vi "HFRR ADV v01.vi"() -> ()   [LabVIEW 2023] (continued)
                n2218 = VISA Write(VISA resource name=w3350, write buffer=w3345, error in (no error)=w3349) -> (VISA resource name out=w3348:refnum<visa-resource-name>, error out=w3347:errorcluster)  [unwired: 1 out]
              }
              frame #1 {
                n2219 = Wait (ms)(milliseconds to wait="wait") -> ()  [unwired: 1 out]
              }
              frame #2 {
                w3355 = FALSE ("Send")
                n2220 = property class="Instr"(reference=w3360, error in=w3359) -> (reference out=w3361:refnum<visa-resource-name>, error out=w3362:errorcluster, "Serial Settings:Number of Bytes at Serial Port"=w3354:u32)
                "Humidity 2" <- w3354
                n2221 = VISA Read(VISA resource name=w3361, byte count=w3354, error in (no error)=w3362) -> (VISA resource name out=w3358:refnum<visa-resource-name>, read buffer=→"Humidity Str Rec":string, error out=w3357:errorcluster)  [unwired: 1 out]
                n2222 = local write "Ser Led"(w3355) -> ()
                n2223 = local write "Send"(w3355) -> ()
              }
            }
            n2224 = Select(t=w3332, s=w3333, f=w3330) -> (s? t:f=w3331:string)
          }
        }
      }
      frame Error {
        w3378 = u16 0 items=["None"=0, "XON/XOFF"=1, "RTS/CTS"=2, "DTR/DSR"=4] ("flow control")
        w3374 = u16 0 items=["None", "Odd", "Even", "Mark", "Space"] ("parity")
        w3377 = u16 10 items=["1.0"=10, "1.5"=15, "2.0"=20] ("stop bits")
        n2225 = VISA Close(VISA resource name=w3370, error in (no error)=w3371) -> (error out=w3369:errorcluster)
        n2226 = local write "Humidity Str Rec"("" ("Humidity Str Rec")) -> ()
        n2227 = call <vilib>:"Clear Errors.vi"("error in (no error)"=w3369) -> ("error out"=w3368:errorcluster)  [unwired: 5 in, 1 out]
        n2228 = local read "Com Port 3"() -> (w3367:refnum<visa-resource-name>)
        n2229 = local write "humid"("" ("humid")) -> ()
        n2230 = call-poly "VISA Configure Serial Port"("VISA resource name"=w3367, "timeout (10sec)"=u32 1000, "termination char\n(0xA = '\\n' = LF)"=u8 10 ("termination char\n(0xA = '\\n' = LF)"), "Enable Termination\nChar (T)"=FALSE ("Enable Termination Char (T)"), "baud rate (9600)"="Humidity BaudRate", "data bits (8)"=u16 8 ("data bits"), "parity (0:none)"=w3374, "error in (no error)"=w3368, "stop bits (10: 1 bit)"=w3377, "flow control (0:none)"=w3378) -> ("VISA resource name out"=w3373:refnum<visa-resource-name>, "error out"=w3364:errorcluster)  [unwired: 4 in]
        "Port 3 Error" <- w3364
      }
    }
    n2231 = local read "Humidity Str Rec"() -> (w3265:string)
    n2232 = String Subset(string=w3265, offset (0)=7) -> (substring=w3280:string)  [unwired: 1 in]
    n2233 = Match Pattern(string=w3280, regular expression="g") -> (after substring=w3281:string, offset past match=w3272:i32)  [unwired: 1 in, 2 out]
    n2234 = Match Pattern(string=w3280, regular expression="y") -> (after substring=w3279:string, offset past match=w3273:i32)  [unwired: 1 in, 2 out]
    n2235 = Match Pattern(string=w3265, regular expression="v") -> (offset past match=w3286:i32)  [unwired: 1 in, 3 out]
    n2236 = Match Pattern(string=w3265, regular expression="?") -> (offset past match=w3283:i32)  [unwired: 1 in, 3 out]
    n2237 = Number To Decimal String(number="Set Rh") -> (decimal integer string=w3290:string)  [unwired: 1 in]
    n2238 = Greater Or Equal To 0?(x=w3273) -> (x >= 0?=w3270:bool)
    n2239 = Greater Or Equal To 0?(x=w3272) -> (x >= 0?=w3271:bool)
    n2240 = Greater Or Equal To 0?(x=w3286) -> (x >= 0?=w3268:bool)
    n2241 = Equal?(x=w3283, y=-1) -> (x = y?=w3267:bool)
    n2242 = Not Equal?(x="Set Rh", y=w3287) -> (x != y?=w3292:bool)
    n2243 = Greater?(x=w3273, y=w3272) -> (0:w3278:bool)
    n2244 = Or(x=w3270, y=w3271) -> (x .or. y?=w3269:bool)
    n2245 = Compound Arithmetic op=AND(w3268, w3267, w3269) -> (w3266:bool)
    n2246 = Concatenate Strings("#setPoint00" ("string"), w3290) -> (w3291:string)
    n2247 = Select(t=w3279, s=w3278, f=w3281) -> (s? t:f=w3274:string)
    n2248 = case shown="True" w3266 {
      tunnel: w3265 -> [_ _]
      tunnel: w3274 -> [_ w3305]
      frame False {
      }
      frame True {
        w3303 = " " ("regular expression")
        n2249 = Match Pattern(string=w3305, regular expression=" ") -> (after substring=w3307:string)  [unwired: 1 in, 3 out]
        n2250 = Match Pattern(string=w3307, regular expression=w3303) -> (before substring=→"humid":string, after substring=w3304:string)  [unwired: 1 in, 2 out]
        n2251 = Match Pattern(string=w3304, regular expression=w3303) -> (before substring=→"temp_@Rh sensor":string)  [unwired: 1 in, 3 out]
      }
    }
    n2252 = case shown="False" w3292 {
      tunnel: w3291 -> [_ w3312]
      frame False {
        n2253 = local read "Rh On/Off"() -> (w3309:bool)
        n2254 = case shown="True" w3309 {
          frame False {
            n2255 = local write "Humidity Str Send"("stop" ("Humidity Str Send")) -> ()
          }
          frame True {
            n2256 = local write "Humidity Str Send"("start" ("Humidity Str Send")) -> ()
          }
        }
      }
      frame True {
        n2257 = local write "Humidity Str Send"(w3312) -> ()
      }
    }
    n2258 = local read "EXIT"() -> (w3293:bool)
  }
  n2259 = VISA Close(VISA resource name=w8, error in (no error)=w9) -> (error out=w19:errorcluster)
  n2260 = call <vilib>:"Clear Errors.vi"("error in (no error)"=w19) -> ()  [unwired: 5 in, 2 out]
  n2261 = Or(x=w21, y=w22) -> (x .or. y?=w20:bool)
  n2262 = Or(x=w46, y=w20) -> (x .or. y?=w45:bool)
  n2263 = while {
    tunnel: [w3387] -> _
    tunnel: w16 -> [_]
    i -> [w3387]
    stop <- w3386 stop-if-true
    # "Langauage selection"
    n2264 = property on="FF Calibration g" class="WFGraph (strict)"("Plot Area:Colors:FG Color"=u32 0) -> ()  [unwired: 2 in, 2 out]
    n2265 = Equal?(x="Lan flag", y=22.0) -> ()  [unwired: 1 out]
    n2266 = case shown="True" "Case Constant\n(See Context Help) 5" {
      frame False {
      }
      frame True {
        n2267 = stacked-sequence {
          frame #0 {
            n2268 = case shown="\"Russian\"" "Language Selection" {
              tunnel: [0 1] -> w3389
              frame "English", Default {
              }
              frame "Russian" {
              }
            }
            n2269 = for {
              N: 130 -> [_]
              tunnel: "Table" -> [w3398]
              tunnel: w3389 -> [w3397]
              i -> [w3396]
              n2270 = Index Array(array=w3398, index (row)=w3396, index (col)=w3397) -> (element=w3395:string)
              n2271 = case shown="8" w3396 {
                tunnel: w3395 -> [w3399 w3400 w3401 w3402 w3403 w3404 w3405 w3406 w3407 w3408 w3409 w3410 w3411 w3412 w3413 w3414 w3415 w3416 w3417 w3418 w3419 w3420 w3421 w3422 w3423 w3424 w3425 w3426 w3427 _ _ w3428 w3429 w3430 w3431 w3432 w3433 w3442 w3449 w3456 w3463 w3467 w3470 w3473 w3475 w3477 w3478 w3479 w3480 w3481 w3482 w3483 w3484 w3485 w3486 w3487 w3488 w3489 w3490 w3491 w3492 w3493 w3494 w3495 w3496 w3497 w3498 w3499 w3500 w3501 w3502 w3503 w3504 w3505 w3506 w3507 w3508 w3509 w3510 w3511 w3512 w3513 w3514 w3515 w3516 w3517 w3518 w3519 w3520 w3521 w3522 w3523 w3524 w3525 w3526 w3527 w3528 w3529 w3530 w3531 w3532 w3533 w3534 w3535 w3536 _ w3537 w3538 w3539 w3540 w3541 w3542 w3543 w3544 w3545 w3546 w3547 w3548 w3549 _ w3550 w3551 w3552 w3553 w3554 w3555 _]
                frame 0 {
                  n2272 = local write "S"(w3399) -> ()
                }
                frame 1 {
                  n2273 = local write "S 2"(w3400) -> ()
                }
                frame 2 {
                  n2274 = property on="EXIT" class="Bool (strict)"("Boolean Text.Text"=w3401) -> ()  [unwired: 2 in, 2 out]
                }
                frame 3 {
                  n2275 = local write "S 4"(w3402) -> ()
                }
                frame 4 {
                  n2276 = property on="FILE" class="Str"("Caption.Text"=w3403) -> ()  [unwired: 2 in, 2 out]
                }
                frame 5 {
                  n2277 = property on="Fuel Discription :" class="Str"("Caption.Text"=w3404) -> ()  [unwired: 2 in, 2 out]
                }
                frame 6 {
                  n2278 = property on="Remarks :" class="Str"("Caption.Text"=w3405) -> ()  [unwired: 2 in, 2 out]
                }
                frame 7 {
                  n2279 = property on="Save & Continue" class="Bool (strict)"("Boolean Text.Text"=w3406) -> ()  [unwired: 2 in, 2 out]
                }
                frame 8 {
                  n2280 = property on="STOP 3" class="Bool (strict)"("Boolean Text.Text"=w3407) -> ()  [unwired: 2 in, 2 out]
                }
                frame 9 {
                  n2281 = property on="Set Hz" class="DigNum (strict)"("Caption.Text"=w3408) -> ()  [unwired: 2 in, 2 out]
                }
                frame 10 {
                  "String 3" <- w3409
                }
                frame 11 {
                  n2282 = property on="NORMAL LOAD" class="DigNum (strict)"("Caption.Text"=w3410) -> ()  [unwired: 2 in, 2 out]
                }
                frame 12 {
                  "String 5" <- w3411
                }
                frame 13 {
                  n2283 = property on="Set Temp" class="DigNum (strict)"("Caption.Text"=w3412) -> ()  [unwired: 2 in, 2 out]
                }
                frame 14 {
                  n2284 = local write "S 15"(w3413) -> ()
                }
                frame 15 {
                  n2285 = property on="Set Rh" class="DigNum (strict)"("Caption.Text"=w3414) -> ()  [unwired: 2 in, 2 out]
                }
                frame 16 {
                  "String 13" <- w3415
                  "String 26" <- w3415
                }
                frame 17 {
                  n2286 = local write "S 18"(w3416) -> ()
                }
                frame 18 {
                  "String 17" <- w3417
                }
                frame 19 {
                  n2287 = property on="test time" class="DigNum (strict)"("Caption.Text"=w3418) -> ()  [unwired: 2 in, 2 out]
                }
                frame 20 {
                  "String 18" <- w3419
                  "String 22" <- w3419
                }
                frame 21 {
                  n2288 = property on="Elapsed time" class="DigNum (strict)"("Caption.Text"=w3420) -> ()  [unwired: 2 in, 2 out]
                }
                frame 22 {
                  n2289 = property on="Samplingtime 2" class="DigNum (strict)"("Caption.Text"=w3421) -> ()  [unwired: 2 in, 2 out]
                }
                frame 23 {
                  "String 21" <- w3422
                }
                frame 24 {
                  n2290 = property on="Countdown" class="DigNum (strict)"("Caption.Text"=w3423) -> ()  [unwired: 2 in, 2 out]
                }
                frame 25 {
                  n2291 = property on="Countdown 2" class="DigNum (strict)"("Caption.Text"=w3424) -> ()  [unwired: 2 in, 2 out]
                }
                frame 26 {
                  n2292 = property on="Engage" class="Bool (strict)"("Boolean Text.Text"=w3425) -> ()  [unwired: 2 in, 2 out]
                }
                frame 27 {
                  n2293 = property on="Boolean  4" class="Bool (strict)"("Boolean Text.Text"=w3426) -> ()  [unwired: 2 in, 2 out]
                }
                frame 28 {
                  n2294 = property on="Test \nStatus" class="Bool (strict)"("Boolean Text.Text"=w3427) -> ()  [unwired: 2 in, 2 out]
                }
                frame 29 {
                }
                frame 30 {
                }
                frame 31 {
                  n2295 = property on="FF Calibration g" class="WFGraph (strict)"("X Scale.Name Label.Text"=w3428) -> ()  [unwired: 2 in, 2 out]
                }
                frame 32 {
                  n2296 = property on="RSTCOF" class="Bool"("Boolean Text.Text"=w3429) -> ()  [unwired: 2 in, 2 out]
                  n2297 = property on="RST FF" class="Bool"("Boolean Text.Text"=w3429) -> ()  [unwired: 2 in, 2 out]
                  n2298 = property on="RST TEMP" class="Bool"("Boolean Text.Text"=w3429) -> ()  [unwired: 2 in, 2 out]
                  n2299 = property on="RSTV1 3" class="Bool"("Boolean Text.Text"=w3429) -> ()  [unwired: 2 in, 2 out]
                  n2300 = property on="rstv2" class="Bool"("Boolean Text.Text"=w3429) -> ()  [unwired: 2 in, 2 out]
                  n2301 = property on="RSTV1 2" class="Bool"("Boolean Text.Text"=w3429) -> ()  [unwired: 2 in, 2 out]
                  n2302 = property on="RST CP" class="Bool"("Boolean Text.Text"=w3429) -> ()  [unwired: 2 in, 2 out]
                }
                frame 33 {
                  "S 61" <- w3430
                }
                frame 34 {
                  "String 23" <- w3431
                }
                frame 35 {
                  n2303 = property on="Rh Before" class="DigNum (strict)"("Caption.Text"=w3432) -> ()  [unwired: 2 in, 2 out]
                }
                frame 36 {
                  n2304 = Match Pattern(string=w3433, regular expression=",") -> (before substring=→"bs":string, after substring=→"as":string)  [unwired: 1 in, 2 out]
                  n2305 = property on="Rh After" class="DigNum (strict)"("Caption.Text"=w3433) -> ()  [unwired: 2 in, 2 out]
                }
                frame 37 {
                  n2306 = Match Pattern(string=w3442, regular expression=",") -> (before substring=w3441:string, after substring=w3440:string)  [unwired: 1 in, 2 out]
                  "bs" <- w3441
                  "as" <- w3440
                  n2307 = Concatenate Strings(w3441, w3440) -> (w3437:string)
                  n2308 = property on="Humidity before test 2" class="DigNum (strict)"("Caption.Text"=w3437) -> ()  [unwired: 2 in, 2 out]
                  n2309 = property on="Humidity before test" class="DigNum (strict)"("Caption.Text"=w3437) -> ()  [unwired: 2 in, 2 out]
                  n2310 = Concatenate Strings(w3437, "=" ("string")) -> (w3438:string)
                  n2311 = local write "S 38"(w3438) -> ()
                }
                frame 38 {
                  n2312 = Match Pattern(string=w3449, regular expression=",") -> (before substring=w3448:string, after substring=w3447:string)  [unwired: 1 in, 2 out]
                  "bs" <- w3448
                  "as" <- w3447
                  n2313 = Concatenate Strings(w3448, w3447) -> (w3444:string)
                  n2314 = property on="Humidity after test 2" class="DigNum (strict)"("Caption.Text"=w3444) -> ()  [unwired: 2 in, 2 out]
                  n2315 = Concatenate Strings(w3444, "=" ("string")) -> (w3446:string)
                  n2316 = property on="Humidity after test" class="DigNum (strict)"("Caption.Text"=w3444) -> ()  [unwired: 2 in, 2 out]
                  n2317 = local write "S 39"(w3446) -> ()
                }
                frame 39 {
                  n2318 = Match Pattern(string=w3456, regular expression=",") -> (before substring=w3455:string, after substring=w3454:string)  [unwired: 1 in, 2 out]
                  "bs" <- w3455
                  "as" <- w3454
                  n2319 = Concatenate Strings(w3455, w3454) -> (w3451:string)
                  n2320 = property on="Temperature before test 2" class="DigNum (strict)"("Caption.Text"=w3451) -> ()  [unwired: 2 in, 2 out]
                  n2321 = property on="Temperature before test" class="DigNum (strict)"("Caption.Text"=w3451) -> ()  [unwired: 2 in, 2 out]
                  n2322 = Concatenate Strings(w3451, "=" ("string")) -> (→"String 34":string)
                }
                frame 40 {
                  n2323 = Match Pattern(string=w3463, regular expression=",") -> (before substring=w3462:string, after substring=w3461:string)  [unwired: 1 in, 2 out]
                  "bs" <- w3462
                  "as" <- w3461
                  n2324 = Concatenate Strings(w3462, w3461) -> (w3458:string)
                  n2325 = property on="Temperature after test 2" class="DigNum (strict)"("Caption.Text"=w3458) -> ()  [unwired: 2 in, 2 out]
                  n2326 = Concatenate Strings(w3458, "=" ("string")) -> (→"String 35":string)
                  n2327 = property on="Temperature after test" class="DigNum (strict)"("Caption.Text"=w3458) -> ()  [unwired: 2 in, 2 out]
                }
                frame 41 {
                  n2328 = property on="AVP" class="DigNum (strict)"("Caption.Text"=w3467) -> ()  [unwired: 2 in, 2 out]
                  n2329 = property on="AVP 2" class="DigNum (strict)"("Caption.Text"=w3467) -> ()  [unwired: 2 in, 2 out]
                  n2330 = Concatenate Strings(w3467, "=" ("string")) -> (→"String 36":string)
                }
                frame 42 {
                  n2331 = property on="MWSD" class="DigNum (strict)"("Caption.Text"=w3470) -> ()  [unwired: 2 in, 2 out]
                  n2332 = property on="MWSD 2" class="DigNum (strict)"("Caption.Text"=w3470) -> ()  [unwired: 2 in, 2 out]
                  n2333 = Concatenate Strings(w3470, "=" ("string")) -> (→"String 37":string)
                }
                frame 43 {
                  n2334 = property on="HCF 2" class="DigNum (strict)"("Caption.Text"=w3473) -> ()  [unwired: 2 in, 2 out]
                  n2335 = property on="HCF" class="DigNum (strict)"("Caption.Text"=w3473) -> ()  [unwired: 2 in, 2 out]
                  n2336 = Concatenate Strings(w3473, "=" ("string")) -> (→"String 38":string)
                }
                frame 44 {
                  n2337 = Concatenate Strings(w3475, "=" ("string")) -> (→"String 39":string)
                  n2338 = property on="WS1.4 2" class="DigNum (strict)"("Caption.Text"=w3475) -> ()  [unwired: 2 in, 2 out]
                  n2339 = property on="WS1.4" class="DigNum (strict)"("Caption.Text"=w3475) -> ()  [unwired: 2 in, 2 out]
                }
                frame 45 {
                  n2340 = property on="Save Results" class="Bool (strict)"("Boolean Text.Text"=w3477) -> ()  [unwired: 2 in, 2 out]
                }
                frame 46 {
                  n2341 = local write "S 47"(w3478) -> ()
                }
                frame 47 {
                  n2342 = local write "S 48"(w3479) -> ()
                }
                frame 48 {
                  n2343 = local write "S 49"(w3480) -> ()
                }
                frame 49 {
                  n2344 = local write "S 50"(w3481) -> ()
                }
                frame 50 {
                  n2345 = local write "S 51"(w3482) -> ()
                }
                frame 51 {
                  n2346 = local write "S 52"(w3483) -> ()
                }
                frame 52 {
                  n2347 = local write "S 53"(w3484) -> ()
                }
                frame 53 {
                  n2348 = local write "S 54"(w3485) -> ()
                }
                frame 54 {
                  n2349 = local write "S 55"(w3486) -> ()
                }
                frame 55 {
                  n2350 = local write "S 56"(w3487) -> ()
                }
                frame 56 {
                  n2351 = local write "S 57"(w3488) -> ()
                }
                frame 57 {
                  n2352 = local write "S 58"(w3489) -> ()
                }
                frame 58 {
                  n2353 = local write "S 59"(w3490) -> ()
                }
                frame 59 {
                  n2354 = local write "S 60"(w3491) -> ()
                }
                frame 60 {
                  n2355 = local write "S 62"(w3492) -> ()
                }
                frame 61 {
                  n2356 = local write "S 63"(w3493) -> ()
                }
                frame 62 {
                  n2357 = local write "S 64"(w3494) -> ()
                }
                frame 63 {
                  n2358 = local write "S 65"(w3495) -> ()
                }
                frame 64 {
                  n2359 = local write "S 66"(w3496) -> ()
                }
                frame 65 {
                  n2360 = local write "S 67"(w3497) -> ()
                }
                frame 66 {
                  n2361 = local write "S 68"(w3498) -> ()
                }
                frame 67 {
                  n2362 = local write "S 69"(w3499) -> ()
                }
                frame 68 {
                  n2363 = local write "S 70"(w3500) -> ()
                }
                frame 69 {
                  n2364 = local write "S 71"(w3501) -> ()
                }
                frame 70 {
                  n2365 = local write "S 72"(w3502) -> ()
                }
                frame 71 {
                  n2366 = local write "S 73"(w3503) -> ()
                }
                frame 72 {
                  n2367 = local write "S 74"(w3504) -> ()
                }
                frame 73 {
                  n2368 = local write "S 75"(w3505) -> ()
                }
                frame 74 {
                  n2369 = local write "S 76"(w3506) -> ()
                }
                frame 75 {
                  n2370 = local write "S 77"(w3507) -> ()
                }
                frame 76 {
                  n2371 = local write "S 78"(w3508) -> ()
                }
                frame 77 {
                  n2372 = local write "S 79"(w3509) -> ()
                }
                frame 79 {
                  n2373 = property on="XY Graph 12" class="XYGraph (strict)"("Y Scale.Name Label.Text"=w3510) -> ()  [unwired: 2 in, 2 out]
                }
                frame 80 {
                  n2374 = local write "S 81"(w3511) -> ()
                  n2375 = property on="XY Graph 11" class="XYGraph (strict)"("Y Scale.Name Label.Text"=w3511) -> ()  [unwired: 2 in, 2 out]
                }
                frame 78 {
                  n2376 = property on="XY Graph 10" class="XYGraph (strict)"("X Scale.Name Label.Text"=w3512) -> ()  [unwired: 2 in, 2 out]
                  n2377 = property on="XY Graph 11" class="XYGraph (strict)"("X Scale.Name Label.Text"=w3512) -> ()  [unwired: 2 in, 2 out]
                  n2378 = property on="XY Graph 12" class="XYGraph (strict)"("X Scale.Name Label.Text"=w3512) -> ()  [unwired: 2 in, 2 out]
                  n2379 = property on="XY Graph 9" class="XYGraph (strict)"("X Scale.Name Label.Text"=w3512) -> ()  [unwired: 2 in, 2 out]
                }
                frame 81 {
                  n2380 = property on="XY Graph 10" class="XYGraph (strict)"("Y Scale.Name Label.Text"=w3513) -> ()  [unwired: 2 in, 2 out]
                }
                frame 82 {
                  n2381 = local write "S 84"(w3514) -> ()
                }
                frame 83 {
                  n2382 = local write "S 85"(w3515) -> ()
                }
                frame 84 {
                  n2383 = local write "S 86"(w3516) -> ()
                }
                frame 85 {
                  n2384 = local write "S 87"(w3517) -> ()
                }
                frame 86 {
                  n2385 = local write "S 88"(w3518) -> ()
                }
                frame 87 {
                  n2386 = property on="FF Calibration g" class="WFGraph (strict)"("Y Scale.Name Label.Text"=w3519) -> ()  [unwired: 2 in, 2 out]
                }
                frame 88 {
                  n2387 = local write "S 90"(w3520) -> ()
                }
                frame 89 {
                  n2388 = local write "S 91"(w3521) -> ()
                }
                frame 90 {
                  n2389 = local write "S 92"(w3522) -> ()
                }
                frame 91 {
                  n2390 = local write "S 93"(w3523) -> ()
                }
                frame 92 {
                  n2391 = local write "S 94"(w3524) -> ()
                }
                frame 93 {
                  n2392 = local write "S 95"(w3525) -> ()
                }
                frame 94 {
                  n2393 = local write "S 96"(w3526) -> ()
                }
                frame 95 {
                  n2394 = local write "S 97"(w3527) -> ()
                }
                frame 96 {
                  n2395 = local write "S 98"(w3528) -> ()
                }
                frame 97 {
                  n2396 = local write "S 99"(w3529) -> ()
                }
                frame 98 {
                  n2397 = local write "S 100"(w3530) -> ()
                }
                frame 99 {
                  n2398 = local write "S 101"(w3531) -> ()
                }
                frame 100 {
                  n2399 = local write "S 102"(w3532) -> ()
                }
                frame 101 {
                  n2400 = local write "S 103"(w3533) -> ()
                }
                frame 102 {
                  n2401 = local write "S 104"(w3534) -> ()
                }
                frame 103 {
                  n2402 = local write "S 105"(w3535) -> ()
                }
                frame 104 {
                  n2403 = local write "S 106"(w3536) -> ()
                }
                frame 105 {
                }
                frame 106 {
                  n2404 = property on="OK Button 17" class="Bool (strict)"("Boolean Text.Text"=w3537) -> ()  [unwired: 2 in, 2 out]
                }
                frame 107 {
                  n2405 = property on="OK Button 16" class="Bool (strict)"("Boolean Text.Text"=w3538) -> ()  [unwired: 2 in, 2 out]
                }
                frame 108 {
                  n2406 = property on="TITTLE" class="Str"("Caption.Text"=w3539) -> ()  [unwired: 2 in, 2 out]
                }
                frame 109 {
                  "String 30" <- w3540
                }
                frame 110 {
                  n2407 = property on="Test Date" class="Str"("Caption.Text"=w3541) -> ()  [unwired: 2 in, 2 out]
                  "String 31" <- w3541
                }
                frame 111 {
                  n2408 = property on="Sample ID" class="Str"("Caption.Text"=w3542) -> ()  [unwired: 2 in, 2 out]
                  "String 32" <- w3542
                }
                frame 112 {
                  n2409 = property on="Tested by" class="Str"("Caption.Text"=w3543) -> ()  [unwired: 2 in, 2 out]
                  "String 33" <- w3543
                }
                frame 113 {
                  n2410 = property on="System Configured Printers 2" class="Arr (strict)"("Caption.Text"=w3544) -> ()  [unwired: 2 in, 2 out]
                }
                frame 114 {
                  n2411 = property on="Selected Printer" class="Str"("Caption.Text"=w3545) -> ()  [unwired: 2 in, 2 out]
                }
                frame 115 {
                  n2412 = property on="Select Printer 3" class="DigNum (strict)"("Caption.Text"=w3546) -> ()  [unwired: 2 in, 2 out]
                }
                frame 116 {
                  n2413 = property on="Print" class="Bool (strict)"("Boolean Text.Text"=w3547) -> ()  [unwired: 2 in, 2 out]
                }
                frame 117 {
                  "String 41" <- w3548
                }
                frame 118 {
                  n2414 = property on="tested by" class="Str"("Caption.Text"=w3549) -> ()  [unwired: 2 in, 2 out]
                }
                frame 119 {
                }
                frame 120 {
                  n2415 = property on="Export" class="Bool (strict)"("Boolean Text.Text"=w3550) -> ()  [unwired: 2 in, 2 out]
                }
                frame 121 {
                  n2416 = property on="TEMP INTERCEPT:" class="DigNum (strict)"("Caption.Text"=w3551) -> ()  [unwired: 2 in, 2 out]
                }
                frame 122 {
                  n2417 = property on="AIR TEMP INTERCEPT:" class="DigNum (strict)"("Caption.Text"=w3552) -> ()  [unwired: 2 in, 2 out]
                }
                frame 123 {
                  n2418 = property on="Select File Type" class="Enum (strict)"("Caption.Text"=w3553) -> ()  [unwired: 2 in, 2 out]
                }
                frame 124 {
                  n2419 = property on="s.NO" class="Str"("Caption.Text"=w3554) -> ()  [unwired: 2 in, 2 out]
                  "String 45" <- w3554
                }
                frame 125 {
                  n2420 = property on="trip1 8" class="Bool (strict)"("Boolean Text.Text"=w3555) -> ()  [unwired: 2 in, 2 out]
                }
                frame 126, Default {
                }
              }
            }
          }
          frame #1 {
            w3563 = TRUE ("Visible")
            n2421 = local read "S 91"() -> (w3580:string)
            n2422 = local read "S 90"() -> (w3579:string)
            n2423 = local read "S 88"() -> (w3578:string)
            n2424 = property on="Threshold" class="DigNum (strict)"("Caption.Text"=w3580) -> ()  [unwired: 2 in, 2 out]
            n2425 = property on="File Path" class="Path"("Caption.Text"=w3579) -> ()  [unwired: 2 in, 2 out]
            n2426 = property on="SrvM CP" class="Bool (strict)"("Boolean Text.Text"=w3578) -> ()  [unwired: 2 in, 2 out]
            n2427 = local read "S 71"() -> (w3573:string)
            n2428 = local read "S 86"() -> (w3575:string)
            n2429 = local read "S 85"() -> (w3576:string)
            n2430 = local read "S 87"() -> (w3574:string)
            n2431 = local read "S 84"() -> (w3577:string)
            n2432 = local read "S 103"() -> (w3562:string)
            n2433 = local read "S 104"() -> (w3561:string)
            n2434 = property on="ENTER THE NEW PASSWORD" class="Str"("Caption.Text"=w3574) -> ()  [unwired: 2 in, 2 out]
            n2435 = property on="Password" class="Str"("Caption.Text"=w3576) -> ()  [unwired: 2 in, 2 out]
            n2436 = property on="ENTER CURRENT PASSWORD" class="Str"("Caption.Text"=w3575) -> ()  [unwired: 2 in, 2 out]
            n2437 = property on="EDIT" class="Bool (strict)"("Boolean Text.Text"=w3573) -> ()  [unwired: 2 in, 2 out]
            n2438 = property on="SAVE" class="Bool (strict)"("Boolean Text.Text"=w3577) -> ()  [unwired: 2 in, 2 out]
            n2439 = Build Array(w3562, w3561) -> (w3560:string[])
            n2440 = property on="Heater Button" class="Bool (strict)"("Strings [4]"=w3560) -> ()  [unwired: 2 in, 2 out]
            n2441 = property on="CH-HUMIDITY WET" class="DigNum (strict)"("Caption.Size to Text?"=w3563) -> ()  [unwired: 2 in, 2 out]
            n2442 = property on="CH-HUMIDITY DRY" class="DigNum (strict)"("Caption.Size to Text?"=w3563) -> ()  [unwired: 2 in, 2 out]
            n2443 = property on="CH-POWER -" class="DigNum (strict)"("Caption.Size to Text?"=w3563) -> ()  [unwired: 2 in, 2 out]
            n2444 = property on="CH-HEATER" class="DigNum (strict)"("Caption.Size to Text?"=w3563) -> ()  [unwired: 2 in, 2 out]
            n2445 = property on="CH-POWER +" class="DigNum (strict)"("Caption.Size to Text?"=w3563) -> ()  [unwired: 2 in, 2 out]
            n2446 = local read "S 92"() -> (w3572:string)
            n2447 = local read "S 93"() -> (w3571:string)
            n2448 = local read "S 105"() -> (w3558:string)
            n2449 = local read "S 106"() -> (w3557:string)
            n2450 = Build Array(w3572, w3571) -> ()  [unwired: 1 out]
            n2451 = Build Array(w3558, w3557) -> (w3559:string[])
            n2452 = local read "S 95"() -> (w3569:string)
            n2453 = local read "S 94"() -> (w3570:string)
            n2454 = local read "bs"() -> (w3585:string)
            n2455 = local read "as"() -> (w3586:string)
            n2456 = property on="Rh On/Off" class="Bool (strict)"("Strings [4]"=w3559) -> ()  [unwired: 2 in, 2 out]
            n2457 = Concatenate Strings(w3585, "\r", w3586) -> ()  [unwired: 1 out]
            n2458 = property on="STROKE GAIN :" class="DigNum (strict)"("Caption.Text"=w3569) -> ()  [unwired: 2 in, 2 out]
            n2459 = property on="DISPLACEMENT :" class="DigNum (strict)"("Caption.Text"=w3570) -> ()  [unwired: 2 in, 2 out]
            n2460 = property on="Rh After" class="DigNum (strict)"("Caption.Size to Text?"=TRUE ("Caption.Size to Text")) -> ()  [unwired: 2 in, 2 out]
            n2461 = local read "S 48"() -> (w3609:string)
            n2462 = local read "S 50"() -> (w3607:string)
            n2463 = local read "S 51"() -> (w3606:string)
            n2464 = local read "S 49"() -> (w3608:string)
            n2465 = local read "S 52"() -> (w3605:string)
            n2466 = local read "as"() -> (w3590:string)
            n2467 = local read "bs"() -> (w3591:string)
            n2468 = local read "S 56"() -> (w3604:string)
            n2469 = local read "S 57"() -> (w3603:string)
            n2470 = local read "S 58"() -> (w3602:string)
            n2471 = local read "S 59"() -> (w3601:string)
            n2472 = property on="OPEN" class="Bool (strict)"("Boolean Text.Text"=w3605) -> ()  [unwired: 2 in, 2 out]
            n2473 = property on="OPEN 1" class="Bool (strict)"("Boolean Text.Text"=w3609) -> ()  [unwired: 2 in, 2 out]
            n2474 = property on="OPEN 2" class="Bool (strict)"("Boolean Text.Text"=w3608) -> ()  [unwired: 2 in, 2 out]
            n2475 = property on="OPEN 3" class="Bool (strict)"("Boolean Text.Text"=w3607) -> ()  [unwired: 2 in, 2 out]
            n2476 = property on="OPEN 4" class="Bool (strict)"("Boolean Text.Text"=w3606) -> ()  [unwired: 2 in, 2 out]
            n2477 = Concatenate Strings(w3591, "\r", w3590) -> ()  [unwired: 1 out]
            n2478 = local read "S 102"() -> (w3564:string)
            n2479 = property on="КОФ1" class="DigNum (strict)"("Caption.Text"=w3604) -> ()  [unwired: 2 in, 2 out]
            n2480 = local read "S 98"() -> (w3568:string)
            n2481 = local read "S 99"() -> (w3567:string)
            n2482 = local read "S 100"() -> (w3566:string)
            n2483 = local read "S 101"() -> (w3565:string)
            n2484 = property on="КОФ2" class="DigNum (strict)"("Caption.Text"=w3603) -> ()  [unwired: 2 in, 2 out]
            n2485 = property on="КОФ3" class="DigNum (strict)"("Caption.Text"=w3602) -> ()  [unwired: 2 in, 2 out]
            n2486 = property on="КОФ4" class="DigNum (strict)"("Caption.Text"=w3601) -> ()  [unwired: 2 in, 2 out]
            n2487 = local read "bs"() -> (w3589:string)
            n2488 = local read "as"() -> (w3588:string)
            n2489 = property on="CH-POWER +" class="DigNum (strict)"("Caption.Text"=w3568) -> ()  [unwired: 2 in, 2 out]
            n2490 = property on="CH-POWER -" class="DigNum (strict)"("Caption.Text"=w3567) -> ()  [unwired: 2 in, 2 out]
            n2491 = property on="CH-HEATER" class="DigNum (strict)"("Caption.Text"=w3566) -> ()  [unwired: 2 in, 2 out]
            n2492 = property on="CH-HUMIDITY DRY" class="DigNum (strict)"("Caption.Text"=w3565) -> ()  [unwired: 2 in, 2 out]
            n2493 = property on="CH-HUMIDITY WET" class="DigNum (strict)"("Caption.Text"=w3564) -> ()  [unwired: 2 in, 2 out]
            n2494 = local read "S 60"() -> (w3600:string)
            n2495 = local read "S 54"() -> (w3610:string)
            n2496 = Concatenate Strings(w3589, "\r", w3588) -> ()  [unwired: 1 out]
            n2497 = Concatenate Strings(w3610, w3600) -> ()  [unwired: 1 out]
            n2498 = local read "S 77"() -> (→"String 43":string)
            n2499 = local read "S 76"() -> (w3583:string)
            n2500 = local read "S 78"() -> (w3582:string)
            n2501 = local read "S 71"() -> (w3594:string)
            n2502 = local read "S 66"() -> (w3599:string)
            n2503 = local read "S 67"() -> (w3598:string)
            n2504 = local read "S 68"() -> (w3597:string)
            n2505 = local read "S 69"() -> (w3596:string)
            n2506 = local read "S 70"() -> (w3595:string)
            n2507 = property on="AIR TEMP" class="DigNum (strict)"("Caption.Text"=w3582) -> ()  [unwired: 2 in, 2 out]
            n2508 = property on="Set Strk" class="DigNum (strict)"("Caption.Text"=w3583) -> ()  [unwired: 2 in, 2 out]
            n2509 = property on="FRIC. FORCE :" class="DigNum (strict)"("Caption.Text"=w3599) -> ()  [unwired: 2 in, 2 out]
            n2510 = property on="TEMPERATURE :" class="DigNum (strict)"("Caption.Text"=w3598) -> ()  [unwired: 2 in, 2 out]
            n2511 = property on="SPEED OUT:" class="DigNum (strict)"("Caption.Text"=w3597) -> ()  [unwired: 2 in, 2 out]
            n2512 = property on="AIR TEMPERATURE :" class="DigNum (strict)"("Caption.Text"=w3596) -> ()  [unwired: 2 in, 2 out]
            n2513 = property on="HUMIDITY:" class="DigNum (strict)"("Caption.Text"=w3595) -> ()  [unwired: 2 in, 2 out]
            n2514 = property on="EDIT" class="Bool (strict)"("Boolean Text.Text"=w3594) -> ()  [unwired: 2 in, 2 out]
            n2515 = local read "S 79"() -> (w3581:string)
            n2516 = property on="Stroke" class="DigNum (strict)"("Caption.Text"=w3581) -> ()  [unwired: 2 in, 2 out]
          }
          frame #2 {
          }
        }
        n2517 = local write "Lan flag"(10.0 ("Lan flag")) -> ()
      }
    }
    n2518 = Wait (ms)(milliseconds to wait=u32 50) -> ()  [unwired: 1 out]
    n2519 = local read "EXIT"() -> (w3386:bool)
  }
  n2520 = flat-sequence {
    tunnel: w43 -> [_]
    frame #0 {
    }
    frame #1 {
      n2521 = Quit LabVIEW(quit? (T)=TRUE) -> ()
      n2522 = local write "EXIT"(FALSE ("EXIT")) -> ()
    }
  }
  n2523 = while {
    tunnel: [w3620] -> w41
    i -> [w3619]
    stop <- w3620 stop-if-true
    n2524 = local read "EXIT"() -> (w3620:bool)
    n2525 = Equal To 0?(x=w3619) -> (x = 0?=w3617:bool)
    n2526 = call "Elapsed Time3"("Time Target (s)"=45.0, "Auto Reset"=TRUE) -> ("Time has Elapsed"=w3616:bool)  [unwired: 10 in, 7 out]
    n2527 = Wait (ms)(milliseconds to wait=u32 50) -> ()  [unwired: 1 out]
    n2528 = Or(x=w3616, y=w3617) -> (x .or. y?=w3618:bool)
    n2529 = case shown="True" w3618 {
      frame False {
      }
      frame True {
        n2530 = call <vilib>:"System Exec.vi"("run minimized? (F)"=TRUE, "error in (no error)"="error in (no error)", "command line"="powercfg.exe -change -monitor-timeout-ac 0") -> ("error out"=w3631:errorcluster)  [unwired: 5 in, 3 out]
        n2531 = call <vilib>:"System Exec.vi"("run minimized? (F)"=TRUE, "error in (no error)"=w3631, "command line"="powercfg.exe -change -disk-timeout-ac 0") -> ("error out"=w3630:errorcluster)  [unwired: 5 in, 3 out]
        n2532 = call <vilib>:"System Exec.vi"("run minimized? (F)"=TRUE, "error in (no error)"=w3630, "command line"="powercfg.exe -change -standby-timeout-ac 0") -> ("error out"=w3629:errorcluster)  [unwired: 5 in, 3 out]
        n2533 = call <vilib>:"System Exec.vi"("run minimized? (F)"=TRUE, "error in (no error)"=w3629, "command line"="powercfg.exe -change -hibernate-timeout-ac 0") -> ("error out"=w3628:errorcluster)  [unwired: 5 in, 3 out]
        n2534 = call <vilib>:"Simple Error Handler.vi"("error in (no error)"=w3628) -> ("error out"=w3634:errorcluster)  [unwired: 4 in, 4 out]
        n2535 = call <vilib>:"Clear Errors.vi"("error in (no error)"=w3634) -> ("error out"=→"error out":errorcluster)  [unwired: 5 in, 1 out]
      }
    }
  }
  n2536 = Compound Arithmetic op=OR(w44, w45, w41) -> (w43:bool)
  n2537 = case shown="True" "Case Constant\n(See Context Help) 6" {
    tunnel: w16 -> [_ w3636]
    frame False {
    }
    frame True {
      n2538 = while {
        tunnel: w3636 -> [_]
        tunnel: [w3637] -> _
        i -> [w3637]
        stop <- w3638 continue-if-true
        n2539 = Wait (ms)(milliseconds to wait=u32 50) -> ()  [unwired: 1 out]
        n2540 = stacked-sequence {
          frame #0 {
            # "Controls Text color"
            # "Controls BG color"
            n2541 = property on="FILE" class="Str"("Text.Text Colors:Text Color"="SC  Text") -> ()  [unwired: 2 in, 2 out]
            n2542 = property on="Fuel Discription :" class="Str"("Text.Text Colors:Text Color"="SC  Text") -> ()  [unwired: 2 in, 2 out]
            n2543 = property on="tested by" class="Str"("Text.Text Colors:Text Color"="SC  Text") -> ()  [unwired: 2 in, 2 out]
            n2544 = property on="Remarks :" class="Str"("Text.Text Colors:Text Color"="SC  Text") -> ()  [unwired: 2 in, 2 out]
            n2545 = property class="DigNum (strict)"("Numeric Text.Text Colors:BG Color"="NC BG") -> ()  [unwired: 2 in, 2 out]
            n2546 = property class="DigNum (strict)"("Numeric Text.Text Colors:BG Color"="NC BG") -> ()  [unwired: 2 in, 2 out]
            n2547 = property class="DigNum (strict)"("Numeric Text.Text Colors:BG Color"="NC BG") -> ()  [unwired: 2 in, 2 out]
            n2548 = property class="DigNum (strict)"("Numeric Text.Text Colors:BG Color"="NC BG") -> ()  [unwired: 2 in, 2 out]
            n2549 = property class="DigNum (strict)"("Numeric Text.Text Colors:BG Color"="NC BG") -> ()  [unwired: 2 in, 2 out]
            n2550 = property class="DigNum (strict)"("Numeric Text.Text Colors:BG Color"="NC BG") -> ()  [unwired: 2 in, 2 out]
            n2551 = property class="DigNum (strict)"("Numeric Text.Text Colors:BG Color"="NC BG") -> ()  [unwired: 2 in, 2 out]
            n2552 = property class="DigNum (strict)"("Numeric Text.Text Colors:BG Color"="NC BG") -> ()  [unwired: 2 in, 2 out]
            n2553 = property class="DigNum (strict)"("Numeric Text.Text Colors:BG Color"="NC BG") -> ()  [unwired: 2 in, 2 out]
            n2554 = property class="DigNum (strict)"("Numeric Text.Text Colors:BG Color"="NC BG") -> ()  [unwired: 2 in, 2 out]
            n2555 = property class="DigNum (strict)"("Numeric Text.Text Colors:BG Color"="NC BG") -> ()  [unwired: 2 in, 2 out]
            n2556 = property class="DigNum (strict)"("Numeric Text.Text Colors:BG Color"="NC BG") -> ()  [unwired: 2 in, 2 out]
            n2557 = property on="FILE" class="Str"("Text.Text Colors:BG Color"="SC BG 3") -> ()  [unwired: 2 in, 2 out]
            n2558 = property on="Fuel Discription :" class="Str"("Text.Text Colors:BG Color"="SC BG 3") -> ()  [unwired: 2 in, 2 out]
            n2559 = property on="tested by" class="Str"("Text.Text Colors:BG Color"="SC BG 3") -> ()  [unwired: 2 in, 2 out]
            n2560 = property on="Remarks :" class="Str"("Text.Text Colors:BG Color"="SC BG 3") -> ()  [unwired: 2 in, 2 out]
            n2561 = property class="DigNum (strict)"("Numeric Text.Text Colors:Text Color"="NC Text") -> ()  [unwired: 2 in, 2 out]
            n2562 = property class="DigNum (strict)"("Numeric Text.Text Colors:Text Color"="NC Text") -> ()  [unwired: 2 in, 2 out]
            n2563 = property class="DigNum (strict)"("Numeric Text.Text Colors:Text Color"="NC Text") -> ()  [unwired: 2 in, 2 out]
            n2564 = property class="DigNum (strict)"("Numeric Text.Text Colors:Text Color"="NC Text") -> ()  [unwired: 2 in, 2 out]
            n2565 = property class="DigNum (strict)"("Numeric Text.Text Colors:Text Color"="NC Text") -> ()  [unwired: 2 in, 2 out]
            n2566 = property class="DigNum (strict)"("Numeric Text.Text Colors:Text Color"="NC Text") -> ()  [unwired: 2 in, 2 out]
            n2567 = property class="DigNum (strict)"("Numeric Text.Text Colors:Text Color"="NC Text") -> ()  [unwired: 2 in, 2 out]
            n2568 = property class="DigNum (strict)"("Numeric Text.Text Colors:Text Color"="NC Text") -> ()  [unwired: 2 in, 2 out]
            n2569 = property class="DigNum (strict)"("Numeric Text.Text Colors:Text Color"="NC Text") -> ()  [unwired: 2 in, 2 out]
            n2570 = property class="DigNum (strict)"("Numeric Text.Text Colors:Text Color"="NC Text") -> ()  [unwired: 2 in, 2 out]
            n2571 = property class="DigNum (strict)"("Numeric Text.Text Colors:Text Color"="NC Text") -> ()  [unwired: 2 in, 2 out]
            n2572 = property class="DigNum (strict)"("Numeric Text.Text Colors:Text Color"="NC Text") -> ()  [unwired: 2 in, 2 out]
            n2573 = property class="DigNum (strict)"("Numeric Text.Text Colors:Text Color"="NI Text  2") -> ()  [unwired: 2 in, 2 out]
            n2574 = property class="DigNum (strict)"("Numeric Text.Text Colors:Text Color"="NI Text  2") -> ()  [unwired: 2 in, 2 out]
            n2575 = property class="DigNum (strict)"("Numeric Text.Text Colors:Text Color"="NI Text  2") -> ()  [unwired: 2 in, 2 out]
            n2576 = property class="DigNum (strict)"("Numeric Text.Text Colors:Text Color"="NI Text  2") -> ()  [unwired: 2 in, 2 out]
            n2577 = property class="DigNum (strict)"("Numeric Text.Text Colors:Text Color"="NI Text  2") -> ()  [unwired: 2 in, 2 out]
            n2578 = property class="DigNum (strict)"("Numeric Text.Text Colors:Text Color"="NI Text  2") -> ()  [unwired: 2 in, 2 out]
            n2579 = property class="DigNum (strict)"("Numeric Text.Text Colors:Text Color"="NI Text  2") -> ()  [unwired: 2 in, 2 out]
            n2580 = property class="DigNum (strict)"("Numeric Text.Text Colors:Text Color"="NI Text  2") -> ()  [unwired: 2 in, 2 out]
            n2581 = property class="DigNum (strict)"("Numeric Text.Text Colors:Text Color"="NI Text  2") -> ()  [unwired: 2 in, 2 out]
            n2582 = property class="DigNum (strict)"("Numeric Text.Text Colors:Text Color"="NI Text  2") -> ()  [unwired: 2 in, 2 out]
            n2583 = property class="DigNum (strict)"("Numeric Text.Text Colors:Text Color"="NI Text  2") -> ()  [unwired: 2 in, 2 out]
            n2584 = property class="DigNum (strict)"("Numeric Text.Text Colors:Text Color"="NI Text  2") -> ()  [unwired: 2 in, 2 out]
            n2585 = property class="DigNum (strict)"("Numeric Text.Text Colors:Text Color"="NI Text  2") -> ()  [unwired: 2 in, 2 out]
            n2586 = property class="DigNum (strict)"("Numeric Text.Text Colors:Text Color"="NI Text  2") -> ()  [unwired: 2 in, 2 out]
            n2587 = property class="DigNum (strict)"("Numeric Text.Text Colors:Text Color"="NI Text  2") -> ()  [unwired: 2 in, 2 out]
            n2588 = property class="DigNum (strict)"("Numeric Text.Text Colors:Text Color"="NI Text  2") -> ()  [unwired: 2 in, 2 out]
            n2589 = property on="XY Graph 9" class="XYGraph (strict)"("Plot Area:Colors:FG Color"="GFG  2", "Plot Area:Colors:BG Color"="GBG   2") -> ()  [unwired: 2 in, 2 out]
            n2590 = property on="XY Graph 11" class="XYGraph (strict)"("Plot Area:Colors:FG Color"="GFG  2", "Plot Area:Colors:BG Color"="GBG   2") -> ()  [unwired: 2 in, 2 out]
            n2591 = property on="XY Graph 10" class="XYGraph (strict)"("Plot Area:Colors:FG Color"="GFG  2", "Plot Area:Colors:BG Color"="GBG   2") -> ()  [unwired: 2 in, 2 out]
            n2592 = property on="XY Graph 12" class="XYGraph (strict)"("Plot Area:Colors:FG Color"="GFG  2", "Plot Area:Colors:BG Color"="GBG   2") -> ()  [unwired: 2 in, 2 out]
            n2593 = property class="DigNum (strict)"("Numeric Text.Text Colors:BG Color"="NI BG 2") -> ()  [unwired: 2 in, 2 out]
            n2594 = property class="DigNum (strict)"("Numeric Text.Text Colors:BG Color"="NI BG 2") -> ()  [unwired: 2 in, 2 out]
            n2595 = property class="DigNum (strict)"("Numeric Text.Text Colors:BG Color"="NI BG 2") -> ()  [unwired: 2 in, 2 out]
            n2596 = property class="DigNum (strict)"("Numeric Text.Text Colors:BG Color"="NI BG 2") -> ()  [unwired: 2 in, 2 out]
            n2597 = property class="DigNum (strict)"("Numeric Text.Text Colors:BG Color"="NI BG 2") -> ()  [unwired: 2 in, 2 out]
            n2598 = property class="DigNum (strict)"("Numeric Text.Text Colors:BG Color"="NI BG 2") -> ()  [unwired: 2 in, 2 out]
            n2599 = property class="DigNum (strict)"("Numeric Text.Text Colors:BG Color"="NI BG 2") -> ()  [unwired: 2 in, 2 out]
            n2600 = property class="DigNum (strict)"("Numeric Text.Text Colors:BG Color"="NI BG 2") -> ()  [unwired: 2 in, 2 out]
            n2601 = property class="DigNum (strict)"("Numeric Text.Text Colors:BG Color"="NI BG 2") -> ()  [unwired: 2 in, 2 out]
            n2602 = property class="DigNum (strict)"("Numeric Text.Text Colors:BG Color"="NI BG 2") -> ()  [unwired: 2 in, 2 out]
            n2603 = property class="DigNum (strict)"("Numeric Text.Text Colors:BG Color"="NI BG 2") -> ()  [unwired: 2 in, 2 out]
            n2604 = property class="DigNum (strict)"("Numeric Text.Text Colors:BG Color"="NI BG 2") -> ()  [unwired: 2 in, 2 out]
            n2605 = property class="DigNum (strict)"("Numeric Text.Text Colors:BG Color"="NI BG 2") -> ()  [unwired: 2 in, 2 out]
            n2606 = property class="DigNum (strict)"("Numeric Text.Text Colors:BG Color"="NI BG 2") -> ()  [unwired: 2 in, 2 out]
            n2607 = property class="DigNum (strict)"("Numeric Text.Text Colors:BG Color"="NI BG 2") -> ()  [unwired: 2 in, 2 out]
            n2608 = property class="DigNum (strict)"("Numeric Text.Text Colors:BG Color"="NI BG 2") -> ()  [unwired: 2 in, 2 out]
            n2609 = property class="Bool"("Colors [4]"="Boolean BC T & BG") -> ()  [unwired: 2 in, 2 out]
            n2610 = property on="Save & Continue" class="Bool (strict)"("Colors [4]"="Boolean BC T & BG") -> ()  [unwired: 2 in, 2 out]
            n2611 = property on="STOP 3" class="Bool (strict)"("Colors [4]"="Boolean BC T & BG") -> ()  [unwired: 2 in, 2 out]
            n2612 = property class="Bool (strict)"("Colors [4]"="Boolean BC T & BG") -> ()  [unwired: 2 in, 2 out]
            n2613 = property class="Bool"("Colors [4]"="Boolean BC T & BG") -> ()  [unwired: 2 in, 2 out]
            n2614 = property class="Bool (strict)"("Colors [4]"="Boolean BC T & BG") -> ()  [unwired: 2 in, 2 out]
            n2615 = property class="Bool (strict)"("Colors [4]"="Boolean BC T & BG") -> ()  [unwired: 2 in, 2 out]
            n2616 = property on="RUN" class="Bool (strict)"("Colors [4]"="Boolean BC T & BG") -> ()  [unwired: 2 in, 2 out]
            n2617 = property class="Bool (strict)"("Colors [4]"="Boolean BC T & BG") -> ()  [unwired: 2 in, 2 out]
            n2618 = property class="Bool"("Colors [4]"="Boolean BC T & BG") -> ()  [unwired: 2 in, 2 out]
            n2619 = property class="Bool (strict)"("Colors [4]"="Boolean BC T & BG") -> ()  [unwired: 2 in, 2 out]
            n2620 = property on="OPEN 1" class="Bool (strict)"("Colors [4]"="Boolean BC T & BG 2") -> ()  [unwired: 2 in, 2 out]
            n2621 = property on="OPEN 2" class="Bool (strict)"("Colors [4]"="Boolean BC T & BG 2") -> ()  [unwired: 2 in, 2 out]
            n2622 = property on="OPEN 3" class="Bool (strict)"("Colors [4]"="Boolean BC T & BG 2") -> ()  [unwired: 2 in, 2 out]
            n2623 = property on="OPEN 4" class="Bool (strict)"("Colors [4]"="Boolean BC T & BG 2") -> ()  [unwired: 2 in, 2 out]
            n2624 = property on="OPEN" class="Bool (strict)"("Colors [4]"="Boolean BC T & BG 2") -> ()  [unwired: 2 in, 2 out]
            n2625 = property on="rstv2" class="Bool"("Colors [4]"="Boolean BC T & BG 2") -> ()  [unwired: 2 in, 2 out]
            n2626 = property on="RST CP" class="Bool"("Colors [4]"="Boolean BC T & BG 2") -> ()  [unwired: 2 in, 2 out]
            n2627 = property on="RSTV1 3" class="Bool"("Colors [4]"="Boolean BC T & BG 2") -> ()  [unwired: 2 in, 2 out]
            n2628 = property on="RSTV1 2" class="Bool"("Colors [4]"="Boolean BC T & BG 2") -> ()  [unwired: 2 in, 2 out]
          }
          frame #1 {
          }
        }
        n2629 = local read "EXIT"() -> (w3638:bool)
      }
    }
  }
  n2630 = case shown="True" "Case Constant\n(See Context Help)" {
    frame False {
    }
    frame True {
      n2631 = while {
        tunnel: [w3886] -> _
        i -> [w3886]
        stop <- w3884 stop-if-true
        n2632 = local read "powstat"() -> (w3883:bool)
        n2633 = case shown="True" w3883 {
          frame False {
          }
          frame True {
            n2634 = local read "RUN"() -> (w3887:bool)
            n2635 = case shown="True" w3887 {
              frame False {
                w3917 = 65.0 ("y")
                n2636 = local read "Set Hz"() -> (w3945:dbl)
                n2637 = local read "NORMAL LOAD"() -> (w3946:dbl)
                n2638 = Multiply(x=w3945, y=60.0) -> (x*y=w3952:dbl)
                n2639 = Multiply(x=1.2 ("y"), y=0.949) -> (x*y=w3921:dbl)
                n2640 = Multiply(x=1.2 ("y"), y=0.8166) -> (x*y=w3925:dbl)
                n2641 = Multiply(x=1.2 ("y"), y=0.851) -> (x*y=w3920:dbl)
                n2642 = local read "FF 2"() -> (w3944:dbl)
                n2643 = Absolute Value(x=w3952) -> (abs(x)=w3950:dbl)
                n2644 = local read "Stroke"() -> (w3919:dbl)
                n2645 = Less?(x=w3919, y=w3925) -> (x < y?=w3922:bool)
                n2646 = In Range and Coerce(upper limit=w3921, x=w3919, lower limit=w3920) -> (In Range?=w3923:bool)  [unwired: 1 out]
                n2647 = case shown="13.." w3944 {
                  tunnel: [1 2 3] -> w3942
                  frame 0..10, Default {
                    # "Normal"
                  }
                  frame 11, 12 {
                  }
                  frame 13.. {
                  }
                }
                "FF STATE" <- w3942
                n2648 = local read "TEMP"() -> (w3905:dbl)
                n2649 = case shown="3601.." w3950 {
                  tunnel: [1 2 3] -> w3948
                  frame 0..3000, Default {
                    # "Normal"
                  }
                  frame 3001..3600 {
                  }
                  frame 3601.. {
                  }
                }
                n2650 = case shown="11.." w3946 {
                  tunnel: [1 3] -> w3947
                  frame 1..10, Default {
                  }
                  frame 11.. {
                  }
                }
                "NL STATE" <- w3947
                n2651 = Multiply(x=1.2 ("y"), y=0.95) -> (x*y=w3935:dbl)
                n2652 = Multiply(x=w3917, y=0.954) -> (x*y=w3909:dbl)
                n2653 = Or(x=w3922, y=w3923) -> (x .or. y?=w3924:bool)
                n2654 = Greater Or Equal?(x=w3919, y=w3935) -> (x >= y?=w3932:bool)
                n2655 = Multiply(x=w3917, y=0.99) -> (x*y=w3906:dbl)
                n2656 = Greater Or Equal?(x=w3905, y=w3906) -> (x >= y?=w3911:bool)
                n2657 = Greater Or Equal?(x=w3905, y=w3909) -> (x >= y?=w3908:bool)
                n2658 = case shown="0, 1, Default" w3919 {
                  tunnel: [1 3] -> w3936
                  frame 0, 1, Default {
                  }
                  frame 2.. {
                  }
                }
                n2659 = case shown="True" w3932 {
                  tunnel: [1 3] -> w3937
                  frame False {
                  }
                  frame True {
                  }
                }
                n2660 = case shown="True" w3924 {
                  tunnel: [1 2] -> w3938
                  frame False {
                  }
                  frame True {
                  }
                }
                n2661 = case shown="..0" w3905 {
                  tunnel: [2 3 3 1] -> w3912
                  frame 61, 62 {
                  }
                  frame 63.. {
